vi "VISATCP通信.vi"   [LabVIEW 2016, in "数据传输系统-06.lvlib"]
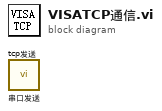
[diagram p0: block diagram]
diagram:
  n1 = call "串口发送.vi"() -> ()  [unwired: 9 in, 3 out]
  n2 = call "tcp发送.vi"() -> ()  [unwired: 9 in, 3 out]
